vi "VI_Solid.vi"() -> ()   [LabVIEW 2017]
uses:
  <vilib>/Motion/Express/_s/nimc.fb.read.readExecutionData.axis.vi
  <vilib>/Motion/Express/_s/nimc.fb.straightLineMove.startStraightLineMove.axis.modeAbsolute.0.vi
  <vilib>/Motion/BlockNode/FB.NIMotion.xnode
  <vilib>/picture/3D Picture Control/NI_3D Picture Control.lvlib
panel:
  out "-x":dbl
  out "output array":dbl[](array[numeric])
  out "3D Picture":refnum<vi>(3d-picture)
  out "Archivos":i32
  in  "Objetos":path
  in  "Mundo":path
  out "Waveform Chart 2":dbl(graph)
  out "Waveform Chart":dbl(graph)
  in  "Stop Button":bool
  out "done":bool
  in  "velocity":dbl=1000.0
  in  "position":dbl=1000.0
  in  "execute":bool
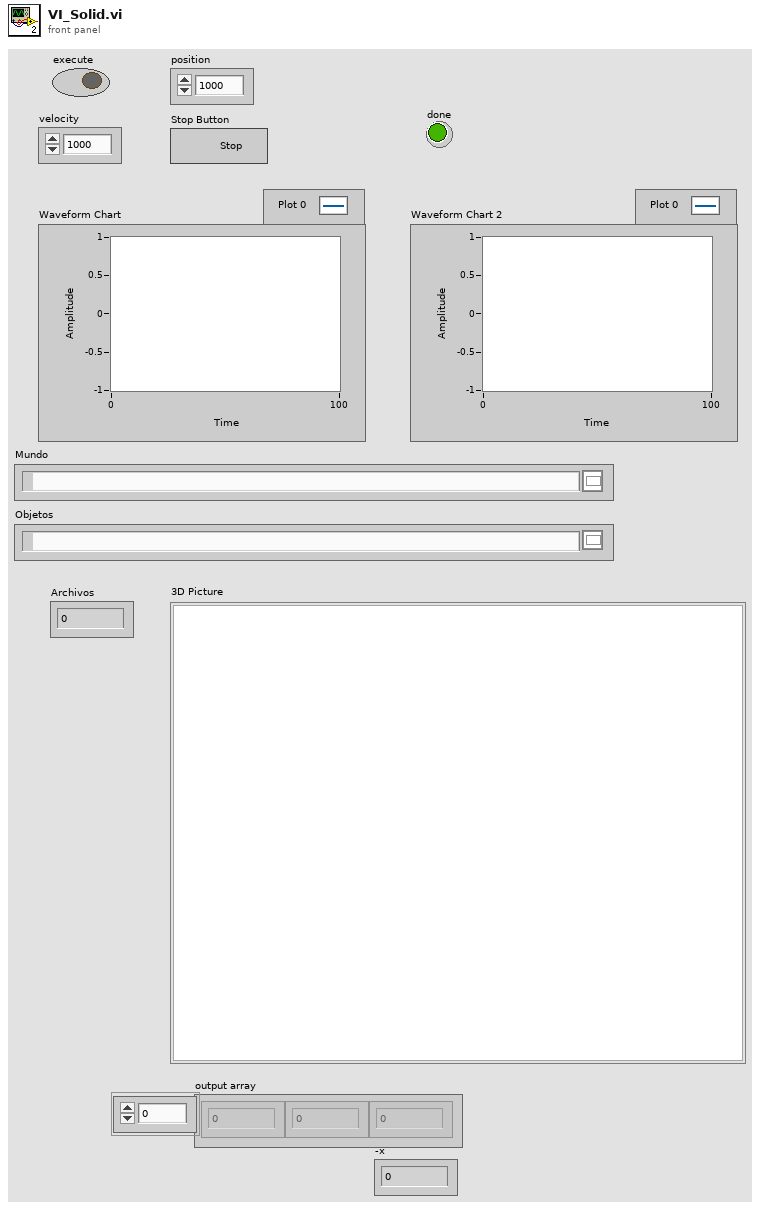
[diagram p1: front panel]
types:
  T1 = enum16{"open", "replace", "create", "open or create", "replace or create", "replace or create with confirmation"}
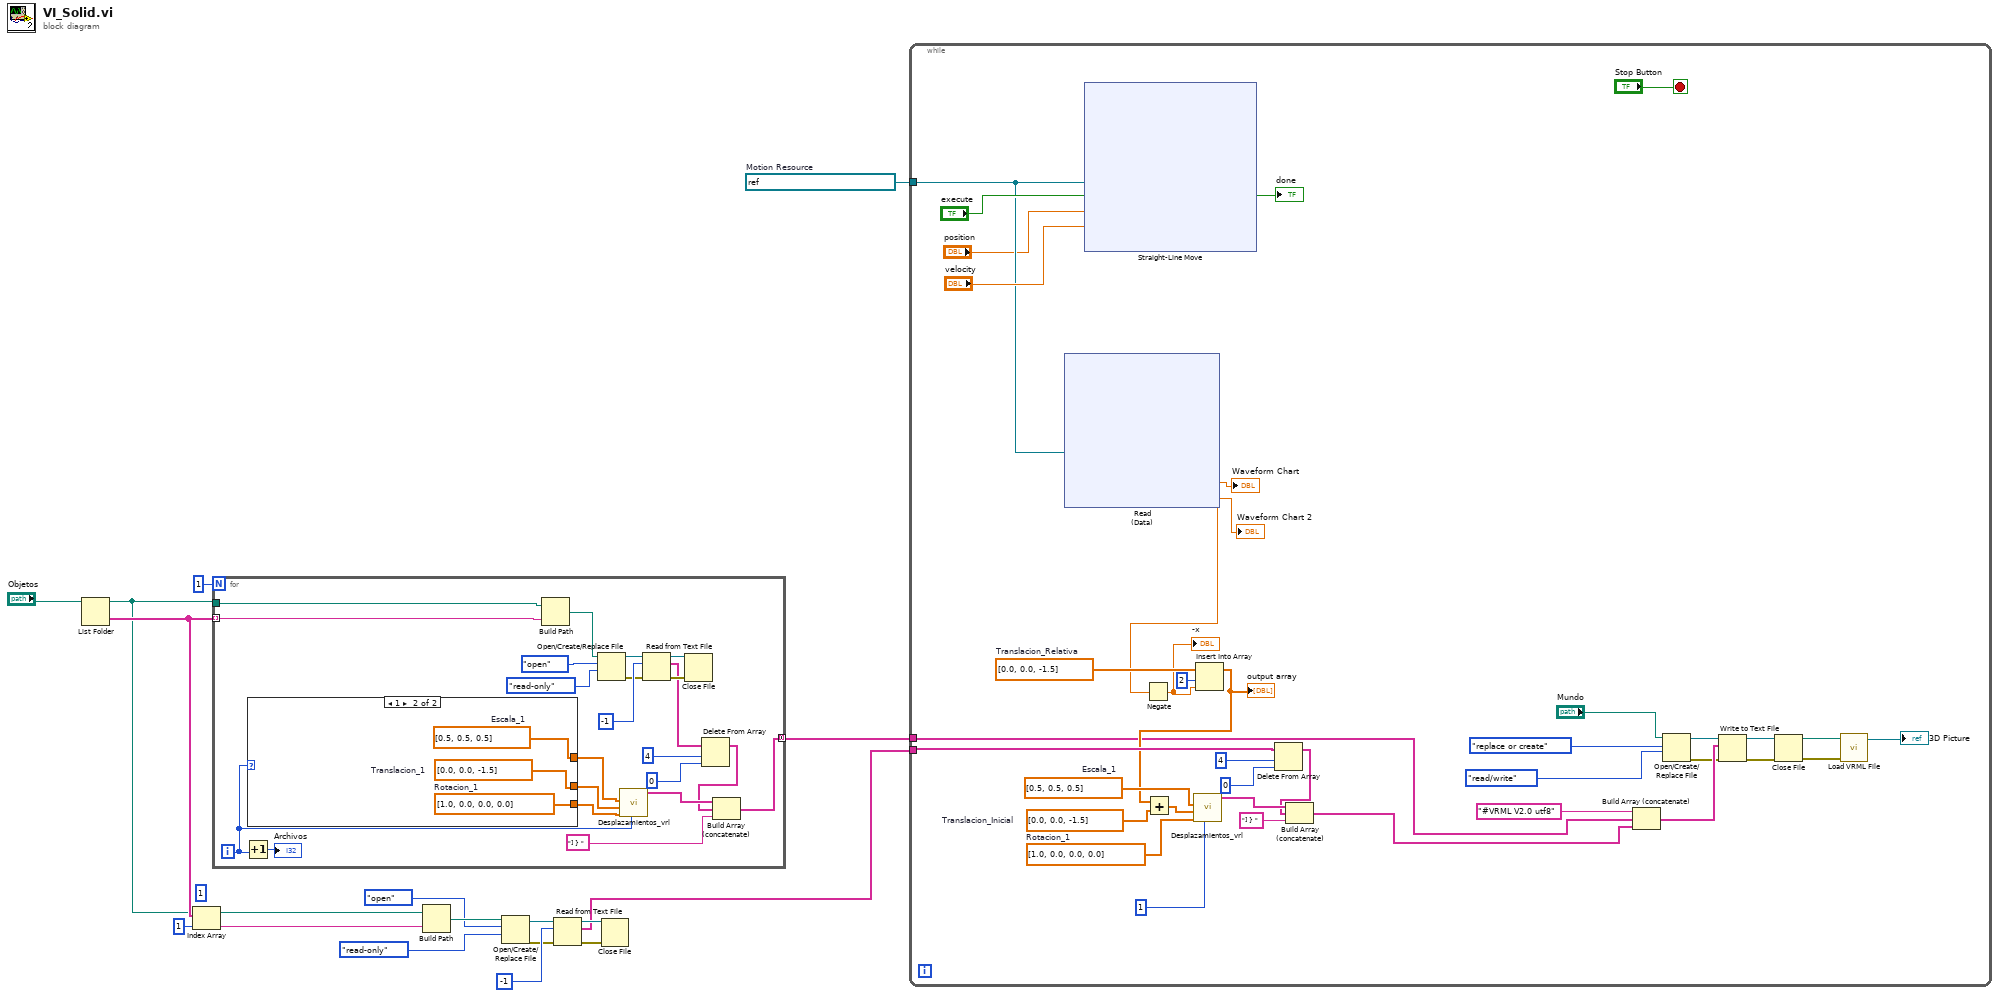
[diagram p0: block diagram]
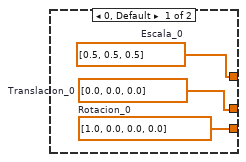
[diagram p2: hidden frame]
diagram:
  (unwired) 1
  w16 = refnum<k21> "nism://My Computer/Eje1"  # Motion Resource
  n1 = List Folder(path="Objetos") -> (filenames=w13:string[])  [unwired: 3 in, 3 out]
  n2 = Index Array(array=w13, index=1) -> (element=w2:string)
  n3 = for {
    N: 1 -> [_]
    tunnel: w13 -> [w38] mode=indexing
    tunnel: "Objetos" -> [w37]
    tunnel: [w25] -> w14 mode=concatenating
    i -> [w17]
    n4 = Increment(x=w17) -> (x+1=→"Archivos":i32)
    n5 = case shown="1" w17 {
      tunnel: [w41 w44] -> w21
      tunnel: [w40 w43] -> w20
      tunnel: [w39 w42] -> w19
      frame 0, Default {
        w41 = dbl[] [1.0, 0.0, 0.0, 0.0]  # Rotacion_0
        w40 = dbl[] [0.0, 0.0, 0.0]  # Translacion_0
        w39 = dbl[] [0.5, 0.5, 0.5]  # Escala_0
      }
      frame 1 {
        w44 = dbl[] [1.0, 0.0, 0.0, 0.0]  # Rotacion_1
        w43 = dbl[] [0.0, 0.0, -1.5]  # Translacion_1
        w42 = dbl[] [0.5, 0.5, 0.5]  # Escala_1
      }
    }
    n6 = Build Path(base path=w37, name or relative path=w38) -> (appended path=w36:path)
    n7 = Open/Create/Replace File(file path (use dialog)=w36, operation (0:open)=T1."open", access (0:read/write)=enum16{"read/write", "read-only", "write-only"}."read-only") -> (refnum out=w33:refnum<file>, error out=w31:errorcluster)  [unwired: 3 in, 1 out]
    n8 = call "Desplazamientos_vrl.vi"("Indice"=w17, "Rotacion"=w21, "Translacion"=w20, "Escala"=w19) -> ("Salida"=w23:string[])  [unwired: 7 in]
    n9 = Read from Text File(file (use dialog)=w33, count=-1, error in=w31) -> (refnum out=w29:refnum<file>, text=w26:string[], error out=w30:errorcluster)  [unwired: 1 in, 1 out]
    n10 = Close File(refnum=w29, error in=w30) -> ()  [unwired: 2 out]
    n11 = Delete From Array(array=w26, length=4, index=0) -> (array with subset deleted=w22:string[])  [unwired: 1 out]
    n12 = Build Array (concatenate)(w23, w22, "] } ") -> (w25:string[])
  }
  n13 = Build Path(base path="Objetos", name or relative path=w2) -> (appended path=w11:path)
  n14 = Open/Create/Replace File(file path (use dialog)=w11, operation (0:open)=T1."open", access (0:read/write)=enum16{"read/write", "read-only", "write-only"}."read-only") -> (refnum out=w8:refnum<file>, error out=w6:errorcluster)  [unwired: 3 in, 1 out]
  n15 = Read from Text File(file (use dialog)=w8, count=-1, error in=w6) -> (refnum out=w4:refnum<file>, text=w1:string[], error out=w5:errorcluster)  [unwired: 1 in, 1 out]
  n16 = Close File(refnum=w4, error in=w5) -> ()  [unwired: 2 out]
  n17 = while {
    tunnel: w16 -> [w77]
    tunnel: w1 -> [w58]
    tunnel: w14 -> [w48]
    stop <- "Stop Button" stop-if-true
    w53 = dbl[] [0.0, 0.0, -1.5]  # Translacion_Relativa
    w55 = dbl[] [1.0, 0.0, 0.0, 0.0]  # Rotacion_1
    w51 = dbl[] [0.0, 0.0, -1.5]  # Translacion_Inicial
    w56 = dbl[] [0.5, 0.5, 0.5]  # Escala_1
    n18 = xnode "Read\n(Data)"("resource"=w77) -> ("position"=w52:dbl, "velocity"=→"Waveform Chart 2":dbl)  [unwired: 1 in, 3 out]
    "Waveform Chart" <- w52
    n19 = xnode "Straight-Line Move"("resource"=w77, "execute"="execute", "position"="position", "velocity"="velocity") -> ("done"=→"done":bool)  [unwired: 2 in, 2 out]
    n20 = Negate(x=w52) -> (-x=w45:dbl)
    "-x" <- w45
    n21 = Insert Into Array(array=w53, index=2, new element=w45) -> (w50:dbl[])
    "output array" <- w50
    n22 = Add(x=w50, y=w51) -> (x+y=w47:dbl[])
    n23 = call "Desplazamientos_vrl.vi"("Indice"=u16 1, "Rotacion"=w55, "Translacion"=w47, "Escala"=w56) -> ("Salida"=w62:string[])  [unwired: 7 in]
    n24 = Delete From Array(array=w58, length=4, index=0) -> (array with subset deleted=w57:string[])  [unwired: 1 out]
    n25 = Build Array (concatenate)(w62, w57, "] } ") -> (w49:string[])
    n26 = Build Array (concatenate)("#VRML V2.0 utf8", w48, w49) -> (w73:string[])
    n27 = Open/Create/Replace File(file path (use dialog)="Mundo", operation (0:open)=T1."replace or create", access (0:read/write)=enum16{"read/write", "read-only", "write-only"}."read/write") -> (refnum out=w67:refnum<file>, error out=w68:errorcluster)  [unwired: 3 in, 1 out]
    n28 = Write to Text File(file (use dialog)=w67, text=w73, error in=w68) -> (refnum out=w70:refnum<file>, error out=w69:errorcluster)  [unwired: 1 in, 1 out]
    n29 = Close File(refnum=w70, error in=w69) -> (path=w71:path, error out=w72:errorcluster)
    n30 = call <vilib>:"Load VRML File.vi"("error in"=w72, "Path"=w71) -> ("Scene:Read Scene File"=→"3D Picture":refnum<vi>)  [unwired: 8 in, 1 out]
  }
